vi "coag pump.vi"(11 "plant flow [L/s]":dbl) -> (0 "In Range?":bool, 1 "coag dose [mg/L]":dbl, 2 "pump [V]":dbl, 3 "coagulant flow [mL/s]":dbl, 5 "rpm":dbl)   [LabVIEW 2015]
uses:
  Sensor buffer command.ctl
  ini.ctl
panel:
  in  "coagulant stock [g/L]":dbl=72.0
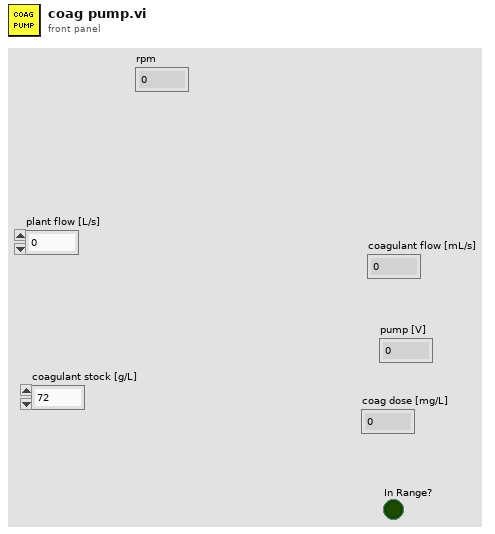
[diagram p1: front panel]
types:
  T1 = typedef "ini.ctl" = enum16{"write", "read"}
  T2 = typedef "Sensor buffer command.ctl" = enum16{"set buffer size", "write", "refill buffer", "read recent", "read all", "clear"}
  T3 = typedef "setpoints.ctl" = cluster{"graph data interval (s)":sgl, "sludge flow [L/s]":dbl, "plant flow [L/s]":dbl, "Plant Flow PID ":cluster{"proportional gain (Kc)":dbl, "integral time (Ti, min)":dbl, "derivative time (Td, min)":dbl}, "Sludge PID ":cluster{"proportional gain (Kc)":dbl, "integral time (Ti, min)":dbl, "derivative time (Td, min)":dbl}, "backwash":T4, "Coagulant":T5}
  T4 = typedef "backwash.ctl" = cluster{"Filtered quality target [NTU]":dbl, "min filtration time [s]":dbl, "Ripen time [s]":dbl}
  T5 = typedef "coag.ctl" = cluster{"flocculator volume (L)":dbl, "clarifier volume (L)":dbl, "dose updates per HRT":u16, "target clarified turbidity (NTU)":dbl, "Coagulant mode":T6, "Coag dose [mg/L]":dbl, "pump mL/rev":dbl, "clarifier flow [L/s]":dbl, "min Coag dose [mg/L]":dbl, "max Coag dose [mg/L]":dbl, "Steps":u16, "HRT response delay":u32, "Ku*":dbl}
  T6 = typedef "model type.ctl" = enum16{"manual", "ramp", "simple corrector", "linear regression"}
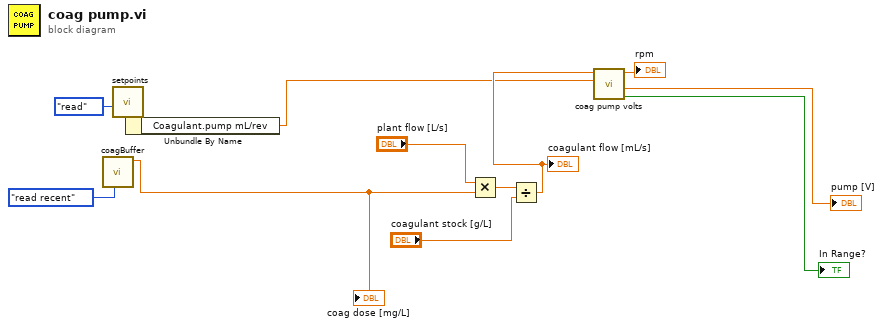
[diagram p0: block diagram]
diagram:
  n1 = call "coagBuffer.vi"("command"=Sensor_buffer_command."read recent") -> ("recent coag"=w9:dbl)  [unwired: 8 in, 2 out]
  "coag dose [mg/L]" <- w9
  n2 = call "setpoints.vi"("ini"=ini."read") -> ("Setpoints out"=w6:T3)  [unwired: 9 in, 1 out]
  n3 = Unbundle By Name(w6) -> ("Coagulant.pump mL/rev"=w4:dbl)
  n4 = Multiply(x="plant flow [L/s]", y=w9) -> (x*y=w11:dbl)
  n5 = Divide(x=w11, y="coagulant stock [g/L]") -> (x/y=w5:dbl)
  "coagulant flow [mL/s]" <- w5
  n6 = call "coag pump volts.vi"("mL/rev"=w4, "coagulant flow [mL/s]"=w5) -> ("In Range?"=→"In Range?":bool, "V"=→"pump [V]":dbl, "rpm"=→"rpm":dbl)  [unwired: 7 in]
